vi "Configure Frequency Sweep.vi"(0 "VISA resource name":refnum<visa-resource-name>, 1 "Enable Frequency Sweep (T: Enable)":bool=TRUE, 5 "Channel (0: Channel 1)":T1 items=["Channel 1", "Channel 2"], 7 "Sweep Spacing (0: Linear)":u16(ring) items=["Linear", "Log"], 9 "Sweep Time (1.00 s)":dbl[unit]=1.0 format="%#.6g", 11 "error in (no error)":errorcluster, 12 "Start Frequency (100 Hz)":dbl[unit]=100.0 format="%#.6g", 13 "Stop  Frequency  (1000 Hz)":dbl[unit]=1000.0 format="%#.6g") -> (4 "VISA resource name out":refnum<visa-resource-name>, 15 "error out":errorcluster)   [LabVIEW 2009, in "Tektronix AFG 3000 Series.lvlib"]
doc: "Configures and enables a frequency sweep. In the frequency sweep mode, the function generator steps from the start frequency to the stop frequency at a sweep rate."
uses:
  Tektronix AFG 3000 Series.lvlib
  controls.llb/Channel.ctl
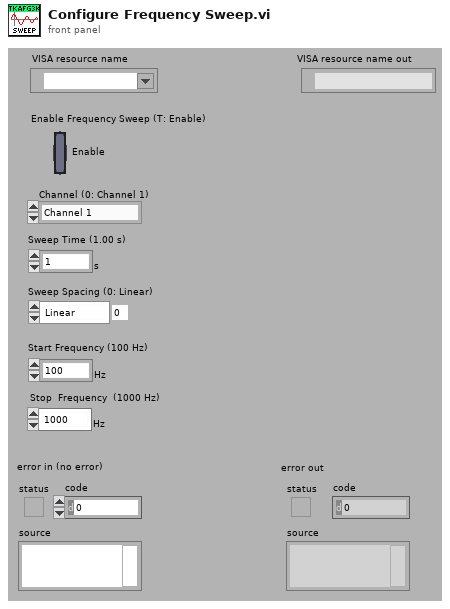
[diagram p1: front panel]
types:
  T1 = typedef "Channel.ctl" = u16
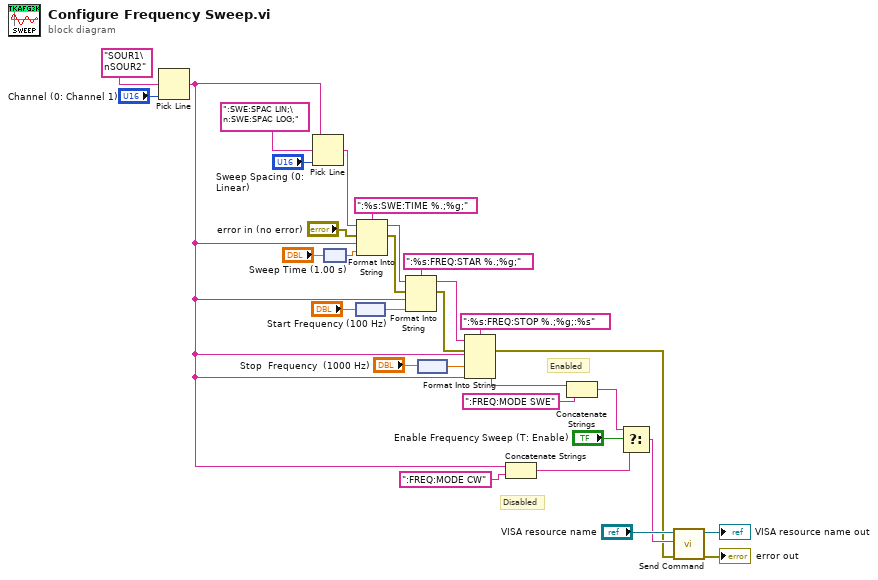
[diagram p0: block diagram]
diagram:
  # "Disabled"
  # "Enabled"
  n1 = Pick Line(multi-line string="SOUR1\nSOUR2" ("string (\"\")"), line index="Channel (0: Channel 1)") -> (output string=w15:string)  [unwired: 1 out]
  n2 = Pick Line(string ("")=w15, multi-line string=":SWE:SPAC LIN;\n:SWE:SPAC LOG;", line index="Sweep Spacing (0: Linear)") -> (output string=w16:string)
  n3 = node("Sweep Time (1.00 s)") -> (w10:dbl)
  n4 = node("Start Frequency (100 Hz)") -> (w8:dbl)
  n5 = Format Into String(format string=":%s:SWE:TIME %.;%g;", initial string=w16, error in="error in (no error)", w15, w10) -> (resulting string=w29:string, error out=w13:errorcluster)
  n6 = Format Into String(format string=":%s:FREQ:STAR %.;%g;", initial string=w29, error in=w13, w15, w8) -> (resulting string=w26:string, error out=w12:errorcluster)
  n7 = node("Stop  Frequency  (1000 Hz)") -> (w6:dbl)
  n8 = Format Into String(format string=":%s:FREQ:STOP %.;%g;:%s", initial string=w26, error in=w12, w15, w6, w15) -> (resulting string=w19:string, error out=w1:errorcluster)
  n9 = Concatenate Strings(w15, ":FREQ:MODE CW" ("Disable")) -> (w20:string)
  n10 = Concatenate Strings(w19, ":FREQ:MODE SWE" ("Enable")) -> (w22:string)
  n11 = Select(t=w22, s="Enable Frequency Sweep (T: Enable)", f=w20) -> (s? t:f=w2:string)
  n12 = call "Send Command.vi"("error in (no error)"=w1, "write buffer"=w2, "VISA resource name"="VISA resource name") -> ("error out"=→"error out":errorcluster, "VISA resource name out"=→"VISA resource name out":refnum<visa-resource-name>)  [unwired: 7 out]
